vi "Finalize Check.vi"(7 "Actor in":refnum<class "Actor.lvclass">, 8 "Error in":errorcluster, 10 "Msg Output":refnum<class "Msg Output.lvclass">) -> (0 "Error out":errorcluster, 2 "Proceed To Tearing Down":bool, 5 "Actor out":refnum<class "Actor.lvclass">)   [LabVIEW 2020, in "jettl.lvlib"]
uses:
  jettl.lvlib
  Actor/Actor.lvclass
  Msg Output/Msg Output.lvclass
  Lifetime.ctl
  Msg/Msg.lvclass
  Stop jettl Msg/Stop/Call.vi
  Stop jettl Msg/Stop/Stop.lvlib
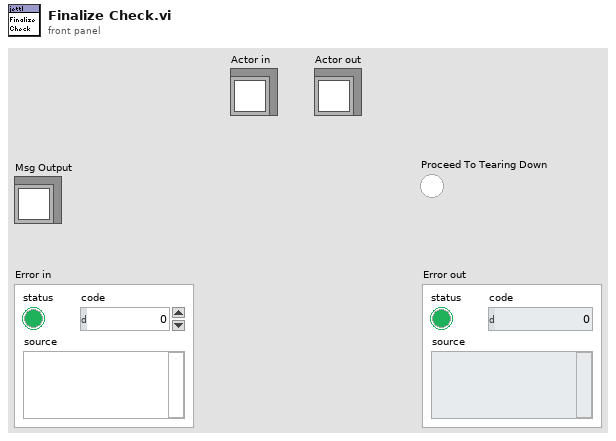
[diagram p1: front panel]
types:
  T1 = typedef "jettl.lvlib/Lifetime.ctl" = enum16{"Init", "Spawn", "Setup", "Teardown Before Started", "Running", "Stopping With Children", "Stopping Without Children", "Teardown After Started", "Stopped"}
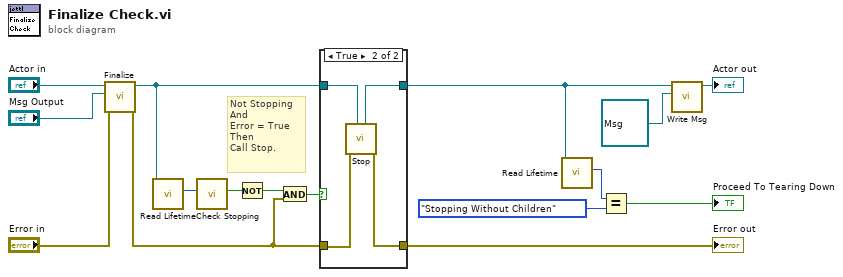
[diagram p0: block diagram]
diagram:
  # "Not Stopping\nAnd\nError = True\nThen\nCall Stop."
  n1 = call-dynamic "Finalize.vi"("Error in"="Error in", "Msg Output"="Msg Output", "Actor in"="Actor in") -> ("Error out"=w5:errorcluster, "Actor out"=w2:refnum<class "Actor.lvclass">)  [unwired: 7 in]
  n2 = call-dynamic "Read Lifetime.vi"("Actor in"=w2) -> ("Lifetime"=w1:T1)  [unwired: 10 in]
  n3 = call "Check Stopping.vi"("Lifetime"=w1) -> ("Stopping"=w4:bool)  [unwired: 10 in]
  n4 = Not(x=w4) -> (.not. x?=w3:bool)
  n5 = And(x=w3, y=w5) -> (x .and. y?=w8:bool)
  n6 = case shown="True" w8 {
    tunnel: [w18 w21] -> w7
    tunnel: w2 -> [w18 w22]
    tunnel: w5 -> [w17 w20]
    tunnel: [w17 w19] -> w6
    frame False {
    }
    frame True {
      n7 = call-poly "Stop.vi"("Actor in"=w22, "Error in"=w20) -> ("Error out"=w19:errorcluster, "Actor out"=w21:refnum<class "Actor.lvclass">)  [unwired: 8 in]
    }
  }
  "Error out" <- w6
  n8 = call-dynamic "Read Lifetime.vi"("Actor in"=w7) -> ("Lifetime"=w13:T1)  [unwired: 10 in]
  n9 = Equal?(x=w13, y=Lifetime."Stopping Without Children") -> (x = y?=→"Proceed To Tearing Down":bool)
  n10 = call-dynamic "Write Msg.vi"("Msg"=refnum<class "Msg.lvclass"> refnum, "Actor in"=w7) -> ("Actor out"=→"Actor out":refnum<class "Actor.lvclass">)  [unwired: 9 in]
